vi "PersistentMaxAndMin.vi"(6 "Reset?":bool, 11 "TimeDomainI":dbl[](array[numeric])) -> (2 "Numeric":dbl, 3 "Numeric 2":dbl)   [LabVIEW 2018]
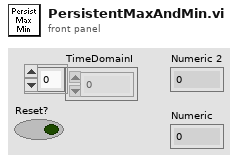
[diagram p1: front panel]
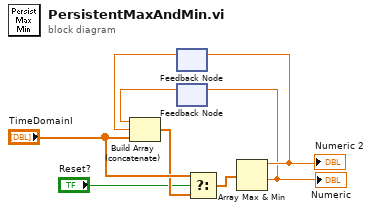
[diagram p0: block diagram]
diagram:
  n1 = feedback #1() -> (w6:dbl)  [unwired: 1 in]
  n2 = feedback #2() -> (w5:dbl)  [unwired: 1 in]
  n3 = Build Array (concatenate)(w5, w6, "TimeDomainI") -> (w2:dbl[])
  n4 = Select(t="TimeDomainI", s="Reset?", f=w2) -> (s? t:f=w3:dbl[])
  n5 = Array Max & Min(array=w3) -> (max value=w8:dbl, min value=w7:dbl)  [unwired: 2 out]
  "Numeric" <- w7
  "Numeric 2" <- w8
  n6 = feedback-in #1(w8) -> ()
  n7 = feedback-in #2(w7) -> ()
